vi "SendCmdToSkywireFixedWait.vi"(6 "wait for response":bool=TRUE, 8 "error in (no error)":errorcluster, 9 "Cmd String":string="AT+CSQ", 10 "Cmd":T1=enum."Get Gemalto model", 11 "VISA resource name":refnum<visa-resource-name>="COM30") -> (0 "error out":errorcluster, 1 "Response numbers":dbl[](array[numeric])=[5.0, 3.0], 2 "Response string":string="AT+CSQ\r\r\n+CSQ: 5,3\r\n\r\nOK\r\n", 3 "VISA resource name 2":refnum<visa-resource-name>="COM30", 4 "Parsed string response":string, 5 "Parsed string responses":string[](array[string]), 7 "RSSI (dbm)":string="-103")   [LabVIEW 2013]
uses:
  Control 1.ctl
  Test Globals/Global 1.vi
  Main Support/Global 2.vi
panel:
  out "Bytes at Port":u32=26
  out "return count":u32=7
  in  "CmdArray":string[](array[string])=["AT+CSQ", "AT+CGMR", "AT+CREG?", "AT+CGREG?", "AT#MEIDESN?", "AT+CGSN", "AT$GPSLOCK?", "In cmd string", "AT", "AT#SIMDET=1", "AT#HDRPS?", "AT+GMM", "AT+KSIMDET=1", "AT#CCID", "AT+CEREG?", "AT+CGMM", "AT+GSN", "AT#SIMDET?"]
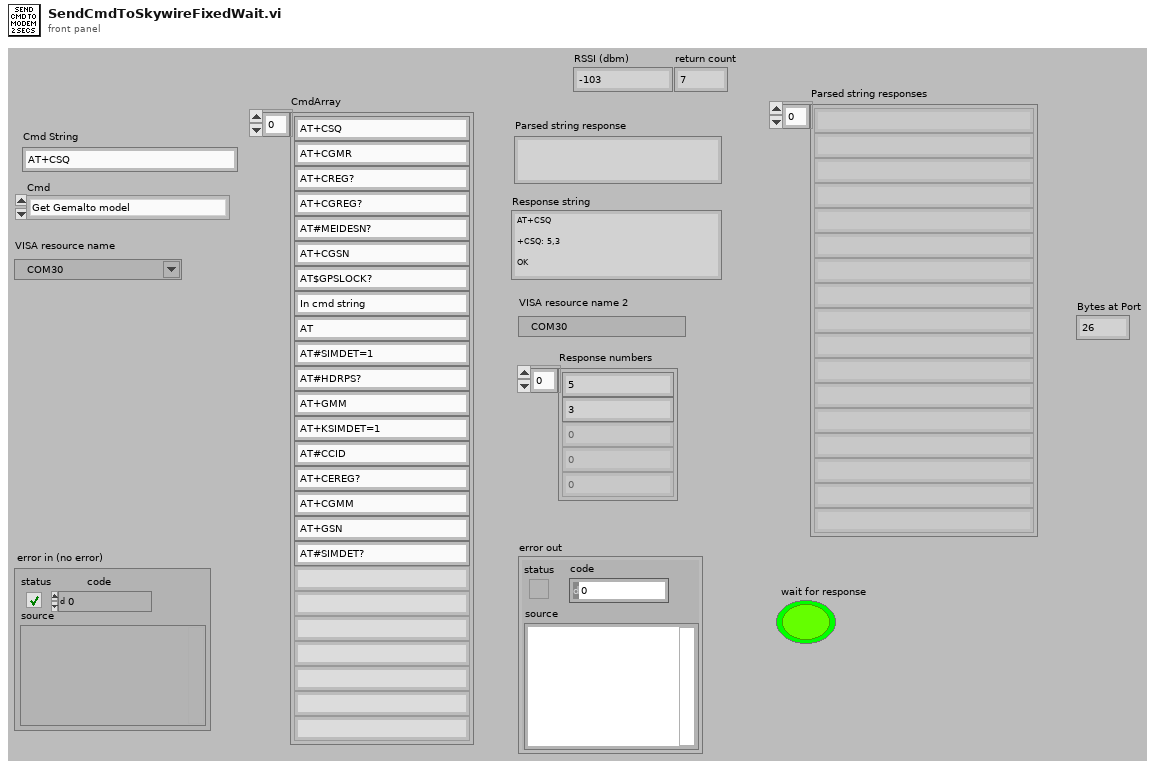
[diagram p1: front panel]
types:
  T1 = typedef "Control 1.ctl" = enum16{"Get primary RSSI", "Get firmware version", "Check 2/3G network reception", "Check LTE network reception", "Get MEID for CDMA", "Get IMEI for 4G/LTE", "Get GPS Coordinates", "Send cmd string", "Check communications", "Enable sim detect", "Check diversity RSSI", "Get make model", "Sierra enable sim det", "get ccid sim id", "Get Gemalto Net Reg", "Get Gemalto model", "Get modem serial number", "Telit sim detect"}
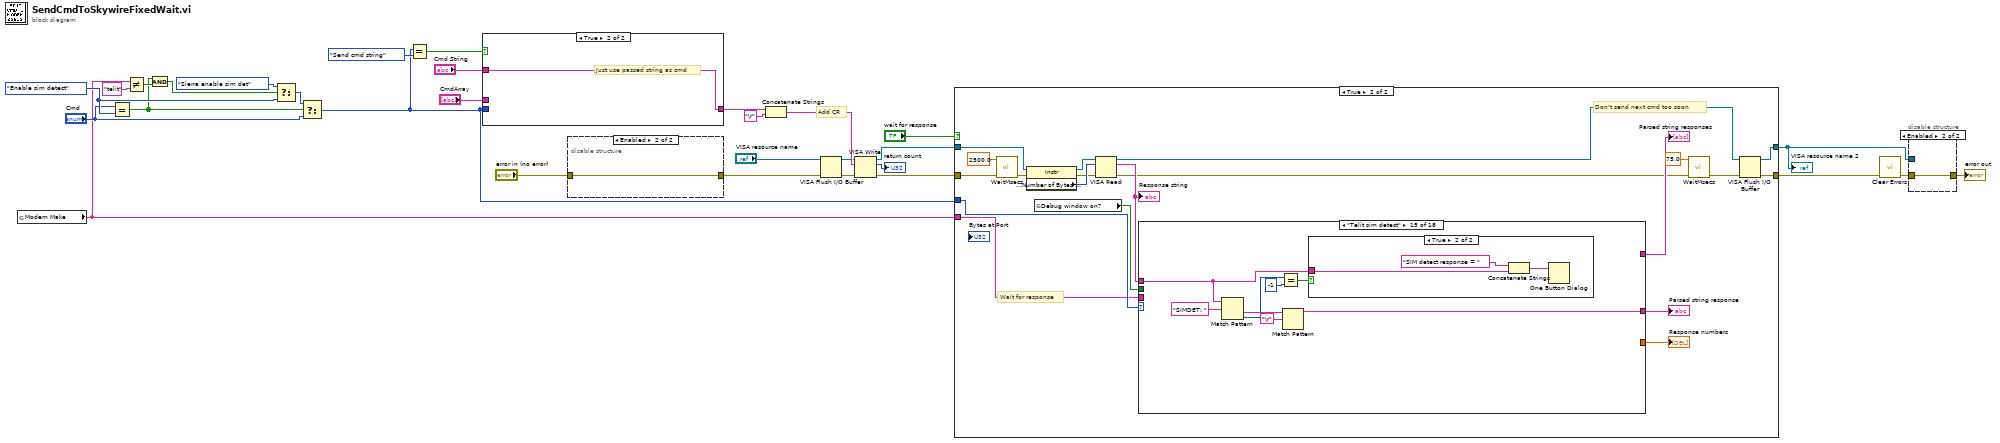
[diagram p0: block diagram]
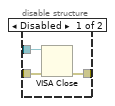
[diagram p2: hidden frame]
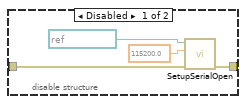
[diagram p3: hidden frame]
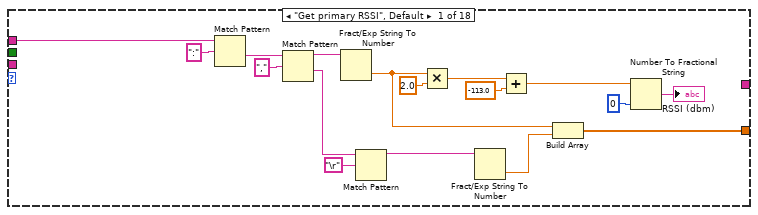
[diagram p5: hidden frame]
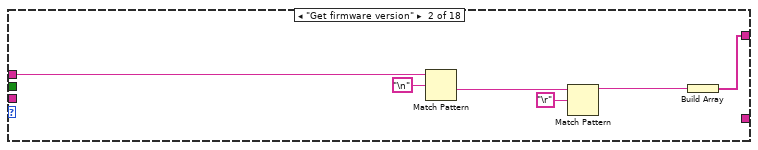
[diagram p6: hidden frame]
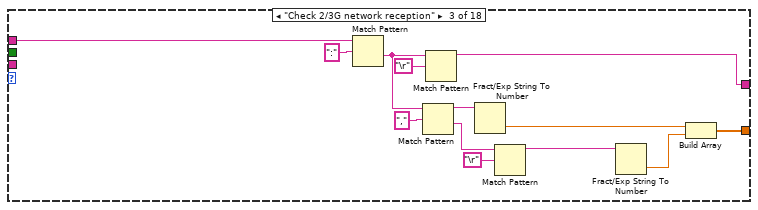
[diagram p7: hidden frame]
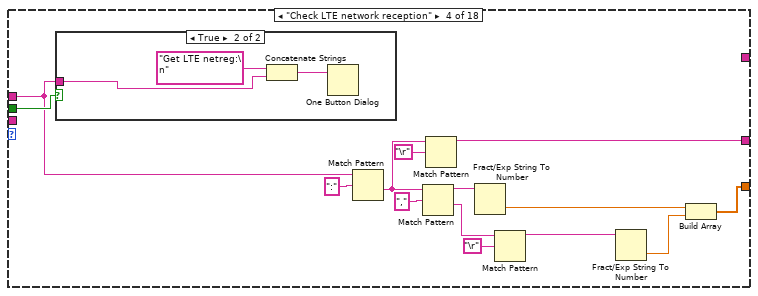
[diagram p8: hidden frame]
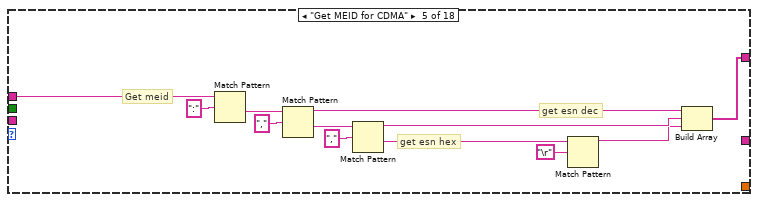
[diagram p10: hidden frame]
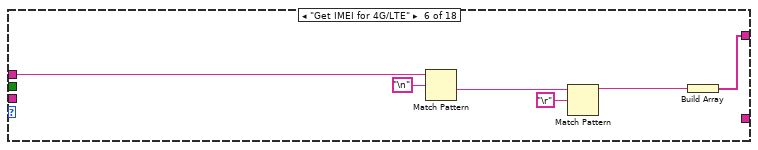
[diagram p11: hidden frame]
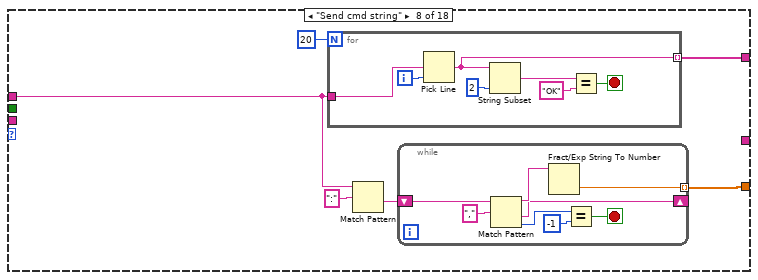
[diagram p13: hidden frame]
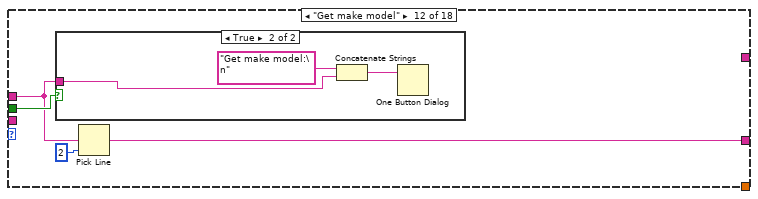
[diagram p17: hidden frame]
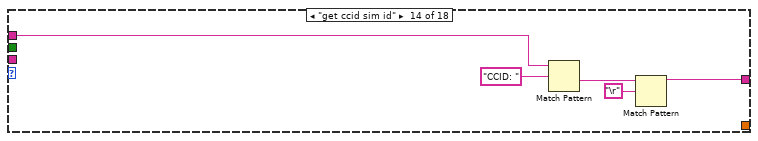
[diagram p20: hidden frame]
diagram:
  w14 = Control_1."Enable sim detect" ("y")
  # "Add CR"
  n1 = global read "Global 1.vi" "Modem Make"() -> (w1:string)
  n2 = Equal?(x="Cmd", y=w14) -> (x = y?=w12:bool)
  n3 = Not Equal?(x=w1, y="telit") -> (x != y?=w17:bool)
  n4 = And(x=w12, y=w17) -> (x .and. y?=w16:bool)
  n5 = Select(t=Control_1."Sierra enable sim det" ("y"), s=w16, f=w14) -> (s? t:f=w13:T1)
  n6 = Select(t=w13, s=w12, f="Cmd") -> (s? t:f=w10:T1)
  n7 = Equal?(x=w10, y=Control_1."Send cmd string") -> (x = y?=w26:bool)
  n8 = case shown="True" w26 {
    tunnel: "CmdArray" -> [w33 _]
    tunnel: [w32 w34] -> w23
    tunnel: "Cmd String" -> [_ w34]
    tunnel: w10 -> [w31 _]
    frame False {
      # "Get cmd string from with cmd as index"
      n9 = Index Array(array=w33, index=w31) -> (element=w32:string)
    }
    frame True {
      # "Just use passed string as cmd"
    }
  }
  n10 = disable-structure shown="Enabled" {
    disable-tunnel: "error in (no error)" -> [w38 w39]
    disable-tunnel: [w37 w39] -> w5
    frame Disabled {
      n11 = call "SetupSerialOpen.vi"("error in (no error)"=w38, "Baud"=115200.0, "VISA Refnum in"=refnum<visa-resource-name> "COM30") -> ("error out"=w37:errorcluster)  [unwired: 7 in, 1 out]
    }
    frame Enabled {
    }
  }
  n12 = Concatenate Strings(w23, "\r") -> (w29:string)
  n13 = VISA Flush I/O Buffer(VISA resource name="VISA resource name", error in (no error)=w5) -> (VISA resource name out=w7:refnum<visa-resource-name>, error out=w9:errorcluster)  [unwired: 1 in]
  n14 = VISA Write(VISA resource name=w7, write buffer=w29, error in (no error)=w9) -> (VISA resource name out=w27:refnum<visa-resource-name>, return count=→"return count":u32, error out=w28:errorcluster)
  n15 = case shown="True" "wait for response" {
    tunnel: [w41 w52] -> w19
    tunnel: w28 -> [w41 w48]
    tunnel: w27 -> [w40 w45]
    tunnel: w10 -> [_ w58]
    tunnel: [w40 w51] -> w2
    tunnel: w1 -> [_ w49]
    frame False {
    }
    frame True {
      # "Don't send next cmd too soon"
      # "Wait for response"
      n16 = call "WaitMsecs.vi"("error in (no error)"=w48, "Wait Msecs"=2500.0) -> ("error out"=w46:errorcluster)  [unwired: 9 in]
      n17 = property class="Instr"(reference=w45, error in=w46) -> (reference out=w44:refnum<visa-resource-name>, error out=w42:errorcluster, "Serial Settings:Number of Bytes at Serial Port"=w43:u32)
      n18 = global read "Global 2.vi" "Debug window on?"() -> (w50:bool)
      n19 = VISA Read(VISA resource name=w44, byte count=w43, error in (no error)=w42) -> (VISA resource name out=w53:refnum<visa-resource-name>, read buffer=w61:string, error out=w54:errorcluster)  [unwired: 1 out]
      "Response string" <- w61
      n20 = case shown="\"Telit sim detect\"" w58 {
        tunnel: w61 -> [w78 w83 w89 w98 w125 w130 _ w134 _ _ _ w154 _ w163 w166 w180 w208 w215]
        tunnel: [w69 _ w88 w103 _ _ _ w136 _ _ _ _ _ _ _ w184 _ _] -> w60
        tunnel: [_ w79 _ _ w115 w127 _ w133 _ _ _ _ _ _ _ _ _ _] -> w59
        tunnel: [_ _ w85 w100 _ _ _ _ _ _ _ w156 _ w161 w170 w177 w210 w216] -> w57
        tunnel: w50 -> [_ _ _ w99 _ _ _ _ _ _ _ w155 _ _ _ _ w209 _]
        tunnel: w49 -> [_ _ _ _ _ _ _ _ _ _ _ _ _ _ _ w183 _ _]
        frame "Get primary RSSI", Default {
          n21 = Match Pattern(string=w78, regular expression=":") -> (after substring=w76:string)  [unwired: 1 in, 3 out]
          n22 = Match Pattern(string=w76, regular expression=",") -> (before substring=w74:string, after substring=w73:string)  [unwired: 1 in, 2 out]
          n23 = Fract/Exp String To Number(string=w74) -> (number=w68:dbl)  [unwired: 3 in, 1 out]
          n24 = Match Pattern(string=w73, regular expression="\r") -> (before substring=w71:string)  [unwired: 1 in, 3 out]
          n25 = Multiply(x=w68, y=2.0) -> (x*y=w66:dbl)
          n26 = Fract/Exp String To Number(string=w71) -> (number=w70:dbl)  [unwired: 3 in, 1 out]
          n27 = Add(x=w66, y=-113.0) -> (x+y=w64:dbl)
          n28 = Build Array(w68, w70) -> (w69:dbl[])
          n29 = Number To Fractional String(number=w64, precision (6)=i16 0) -> (F-format string=→"RSSI (dbm)":string)  [unwired: 2 in]
        }
        frame "Get firmware version" {
          n30 = Match Pattern(string=w83, regular expression="\n") -> (after substring=w84:string)  [unwired: 1 in, 3 out]
          n31 = Match Pattern(string=w84, regular expression="\r") -> (before substring=w80:string)  [unwired: 1 in, 3 out]
          n32 = Build Array(w80) -> (w79:string[])
        }
        frame "Check 2/3G network reception" {
          n33 = Match Pattern(string=w89, regular expression=":") -> (after substring=w86:string)  [unwired: 1 in, 3 out]
          n34 = Match Pattern(string=w86, regular expression=",") -> (before substring=w95:string, after substring=w94:string)  [unwired: 1 in, 2 out]
          n35 = Match Pattern(string=w86, regular expression="\r") -> (before substring=w85:string)  [unwired: 1 in, 3 out]
          n36 = Fract/Exp String To Number(string=w95) -> (number=w91:dbl)  [unwired: 3 in, 1 out]
          n37 = Match Pattern(string=w94, regular expression="\r") -> (before substring=w92:string)  [unwired: 1 in, 3 out]
          n38 = Fract/Exp String To Number(string=w92) -> (number=w90:dbl)  [unwired: 3 in, 1 out]
          n39 = Build Array(w91, w90) -> (w88:dbl[])
        }
        frame "Check LTE network reception" {
          n40 = case shown="True" w99 {
            tunnel: w98 -> [_ w112]
            frame False {
            }
            frame True {
              n41 = Concatenate Strings("Get LTE netreg:\n" ("string"), w112) -> (w113:string)
              n42 = One Button Dialog(message=w113) -> ()  [unwired: 1 in, 1 out]
            }
          }
          n43 = Match Pattern(string=w98, regular expression=":") -> (after substring=w101:string)  [unwired: 1 in, 3 out]
          n44 = Match Pattern(string=w101, regular expression=",") -> (before substring=w109:string, after substring=w108:string)  [unwired: 1 in, 2 out]
          n45 = Match Pattern(string=w101, regular expression="\r") -> (before substring=w100:string)  [unwired: 1 in, 3 out]
          n46 = Fract/Exp String To Number(string=w109) -> (number=w105:dbl)  [unwired: 3 in, 1 out]
          n47 = Match Pattern(string=w108, regular expression="\r") -> (before substring=w106:string)  [unwired: 1 in, 3 out]
          n48 = Fract/Exp String To Number(string=w106) -> (number=w104:dbl)  [unwired: 3 in, 1 out]
          n49 = Build Array(w105, w104) -> (w103:dbl[])
        }
        frame "Get MEID for CDMA" {
          # "get esn hex"
          # "get esn dec"
          # "Get meid"
          n50 = Match Pattern(string=w125, regular expression=":") -> (after substring=w126:string)  [unwired: 1 in, 3 out]
          n51 = Match Pattern(string=w126, regular expression=",") -> (before substring=w120:string, after substring=w121:string)  [unwired: 1 in, 2 out]
          n52 = Match Pattern(string=w121, regular expression=",") -> (before substring=w119:string, after substring=w118:string)  [unwired: 1 in, 2 out]
          n53 = Match Pattern(string=w118, regular expression="\r") -> (before substring=w116:string)  [unwired: 1 in, 3 out]
          n54 = Build Array(w120, w119, w116) -> (w115:string[])
        }
        frame "Get IMEI for 4G/LTE" {
          n55 = Match Pattern(string=w130, regular expression="\n") -> (after substring=w132:string)  [unwired: 1 in, 3 out]
          n56 = Match Pattern(string=w132, regular expression="\r") -> (before substring=w128:string)  [unwired: 1 in, 3 out]
          n57 = Build Array(w128) -> (w127:string[])
        }
        frame "Get GPS Coordinates" {
        }
        frame "Send cmd string" {
          n58 = for {
            N: 20 -> [_]
            tunnel: w134 -> [w145]
            tunnel: [w142] -> w133 mode=indexing
            i -> [w144]
            stop <- w143 stop-if-true
            n59 = Pick Line(multi-line string=w145, line index=w144) -> (output string=w142:string)  [unwired: 1 in]
            n60 = String Subset(string=w142, length (rest)=2 ("length (rest)")) -> (substring=w140:string)  [unwired: 1 in]
            n61 = Equal?(x=w140, y="OK") -> (x = y?=w143:bool)
          }
          n62 = Match Pattern(string=w134, regular expression=":") -> (after substring=w138:string)  [unwired: 1 in, 3 out]
          n63 = while {
            shift-right: [w147] -> _
            shift-left: w138 -> [w151]
            tunnel: [w146] -> w136 mode=indexing
            stop <- w148 stop-if-true
            n64 = Match Pattern(string=w151, regular expression=",") -> (before substring=w153:string, after substring=w147:string, offset past match=w150:i32)  [unwired: 1 in, 1 out]
            n65 = Fract/Exp String To Number(string=w153) -> (number=w146:dbl)  [unwired: 3 in, 1 out]
            n66 = Equal?(x=w150, y=-1) -> (x = y?=w148:bool)
          }
        }
        frame "Check communications" {
        }
        frame "Enable sim detect" {
        }
        frame "Check diversity RSSI" {
        }
        frame "Get make model" {
          n67 = case shown="True" w155 {
            tunnel: w154 -> [_ w158]
            frame False {
            }
            frame True {
              n68 = Concatenate Strings("Get make model:\n" ("string"), w158) -> (w159:string)
              n69 = One Button Dialog(message=w159) -> ()  [unwired: 1 in, 1 out]
            }
          }
          n70 = Pick Line(multi-line string=w154, line index=2) -> (output string=w156:string)  [unwired: 1 in]
        }
        frame "Sierra enable sim det" {
        }
        frame "get ccid sim id" {
          n71 = Match Pattern(string=w163, regular expression="CCID: ") -> (after substring=w162:string)  [unwired: 1 in, 3 out]
          n72 = Match Pattern(string=w162, regular expression="\r") -> (before substring=w161:string)  [unwired: 1 in, 3 out]
        }
        frame "Telit sim detect" {
          n73 = Match Pattern(string=w166, regular expression="SIMDET: ") -> (after substring=w171:string, offset past match=w169:i32)  [unwired: 1 in, 2 out]
          n74 = Equal?(x=w169, y=-1) -> (x = y?=w167:bool)
          n75 = Match Pattern(string=w171, regular expression="\r") -> (before substring=w170:string)  [unwired: 1 in, 3 out]
          n76 = case shown="True" w167 {
            tunnel: w166 -> [_ w174]
            frame False {
            }
            frame True {
              n77 = Concatenate Strings("SIM detect response = " ("string"), w174) -> (w176:string)
              n78 = One Button Dialog(message=w176) -> ()  [unwired: 1 in, 1 out]
            }
          }
        }
        frame "Get Gemalto Net Reg" {
          n79 = Equal?(x=w183, y="wnc") -> (x = y?=w181:bool)
          n80 = case shown="True" w181 {
            tunnel: w180 -> [w189 w202]
            tunnel: [w186 w200] -> w179
            tunnel: [w185 w199] -> w178
            tunnel: [w187 w197] -> w177
            frame False {
              n81 = Match Pattern(string=w189, regular expression=":") -> (after substring=w196:string)  [unwired: 1 in, 3 out]
              n82 = Match Pattern(string=w196, regular expression=",") -> (before substring=w191:string, after substring=w192:string)  [unwired: 1 in, 2 out]
              n83 = Match Pattern(string=w196, regular expression="\r") -> (before substring=w187:string)  [unwired: 1 in, 3 out]
              n84 = Fract/Exp String To Number(string=w191) -> (number=w185:dbl)  [unwired: 3 in, 1 out]
              n85 = Match Pattern(string=w192, regular expression="\r") -> (before substring=w194:string)  [unwired: 1 in, 3 out]
              n86 = Fract/Exp String To Number(string=w194) -> (number=w186:dbl)  [unwired: 3 in, 1 out]
            }
            frame True {
              w201 = "," ("regular expression")
              n87 = Match Pattern(string=w202, regular expression=":") -> (after substring=w207:string)  [unwired: 1 in, 3 out]
              n88 = Match Pattern(string=w207, regular expression=w201) -> (before substring=w203:string, after substring=w204:string)  [unwired: 1 in, 2 out]
              n89 = Match Pattern(string=w207, regular expression="\r") -> (before substring=w197:string)  [unwired: 1 in, 3 out]
              n90 = Fract/Exp String To Number(string=w203) -> (number=w199:dbl)  [unwired: 3 in, 1 out]
              n91 = Match Pattern(string=w204, regular expression=w201) -> (before substring=w205:string)  [unwired: 1 in, 3 out]
              n92 = Fract/Exp String To Number(string=w205) -> (number=w200:dbl)  [unwired: 3 in, 1 out]
            }
          }
          n93 = Build Array(w178, w179) -> (w184:dbl[])
        }
        frame "Get Gemalto model" {
          n94 = case shown="True" w209 {
            tunnel: w208 -> [_ w213]
            frame False {
            }
            frame True {
              n95 = Concatenate Strings("Gemalto model = " ("string"), w213) -> (w212:string)
              n96 = One Button Dialog(message=w212) -> ()  [unwired: 1 in, 1 out]
            }
          }
          n97 = Pick Line(multi-line string=w208, line index=2) -> (output string=w210:string)  [unwired: 1 in]
        }
        frame "Get modem serial number" {
          n98 = Pick Line(multi-line string=w215, line index=2) -> (output string=w216:string)  [unwired: 1 in]
        }
      }
      "Response numbers" <- w60
      "Parsed string response" <- w57
      "Parsed string responses" <- w59
      n99 = call "WaitMsecs.vi"("error in (no error)"=w54, "Wait Msecs"=75.0) -> ("error out"=w56:errorcluster)  [unwired: 9 in]
      n100 = VISA Flush I/O Buffer(VISA resource name=w53, error in (no error)=w56) -> (VISA resource name out=w51:refnum<visa-resource-name>, error out=w52:errorcluster)  [unwired: 1 in]
    }
  }
  "VISA resource name 2" <- w2
  n101 = call <vilib>:"Clear Errors.vi"("error in (no error)"=w19) -> ("error out"=w4:errorcluster)  [unwired: 6 in]
  n102 = disable-structure shown="Enabled" {
    disable-tunnel: w4 -> [w220 w221]
    disable-tunnel: [w219 w221] -> w3
    disable-tunnel: w2 -> [w218 _]
    frame Disabled {
      n103 = VISA Close(VISA resource name=w218, error in (no error)=w220) -> (error out=w219:errorcluster)
    }
    frame Enabled {
    }
  }
  "error out" <- w3
